vi "{TMPL} MAIN - App.vi"() -> ()   [LabVIEW 2023, in "TLB` InstStu GPlugin Template.lvlib" / "{TMPL} TLB`.lvclass"]
uses:
  {TMPL} TLB`.lvclass
  Application Components/Trigger API/System Trigger.ctl
  State Machine/State.ctl
  Core Components/Error Handler/TLB` Error Handler.lvclass
  Application Components/Configuration/{TMPL} Station Configuration.lvclass
  {TMPL} TLB`.lvclass/{TMPL} TLB`.ctl
  <vilib>/Utility/error.llb/Error Cluster From Error Code.vi
  <vilib>/ErrorRing/Error Ring.xnode
  Application Components/Trigger API/{TMPL} Trigger API.lvlib
  TLB` InstStu GPlugin Template.lvlib
  Core Components/Actions/Actions.lvlib
  Core Components/Dependencies/TLB`_Dependencies.lvlib
panel:
  out "top banner":u32(colorbox)=44412
  out "iq graph":waveform(sgl)[](graph) caption="Q Data"
  out "iq graph 2":waveform(sgl)[](graph) caption="Q Data"
  out "iq graph 3":waveform(sgl)[](graph) caption="Q Data"
  out "iq graph 4":waveform(sgl)[](graph) caption="Q Data"
  in  "error":bool
  out "error background":u32(colorbox)=15461355
  in  "settings gear":bool
  in  "connect":bool
  in  "run":bool
  in  "single":bool
  out "title":string="INST STU GPLUGIN`"
  in  "INSTRUMENT":refnum<visa-resource-name>
  out "error out":errorcluster
  in  "digital offset":dbl caption="DIGITAL OFFSET" format="%1_3p"
  in  "digital gain":dbl=-10.0 caption="DIGITAL GAIN" format="%1_3p dB"
  in  "finite records?":bool=TRUE
  in  "iq rate":dbl=2160000000.0 caption="IQ  RATE" format="%1_6p samples/sec"
  in  "no of samples":u64=1000 caption="NO. SAMPLES"
  in  "no of records":u64=25 caption="NO. RECORDS"
  in  "finite samples?":bool=TRUE
  in  "acq sample rate":dbl=2160000000.0 caption="ACQ SAMPLE RATE" format="%1_6p samples/sec"
  out "State":string="<Shutdown> "
  out "Status":string
  # "Section  A"
  # "Section B"
  # "Category A"
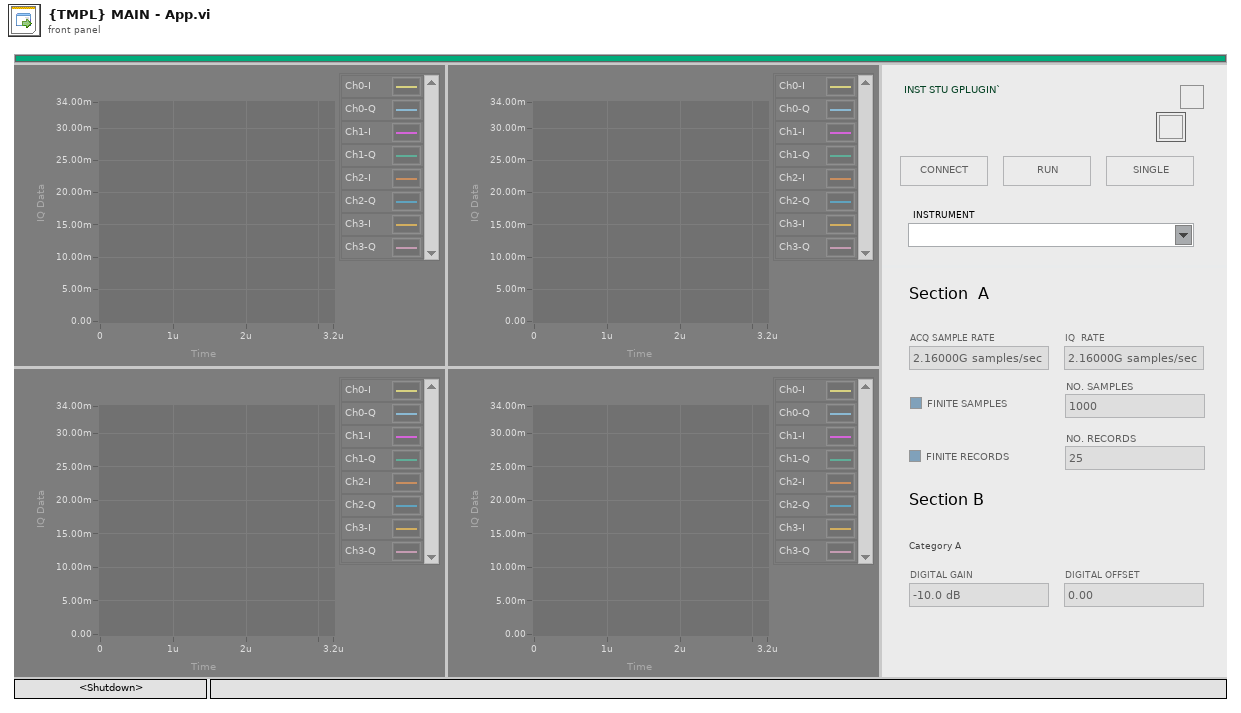
[diagram p1: front panel]
types:
  T1 = typedef "TLB` InstStu GPlugin Template.lvlib/{TMPL} TLB`.lvclass/State.ctl" = enum16{"<Startup>", "Idle", "Connected", "Monitoring", "<Shutdown>", "<Error>"}
  T2 = enum16{"Close Display", "Clear References", "Close Error Handler"}
  T3 = enum16{"Clear SR", "Set Display", "Set Shifter", "Initialize Events", "Init Q"}
  T4 = typedef "TLB` InstStu GPlugin Template.lvlib/{TMPL} Trigger API.lvlib/System Trigger.ctl" = enum16{"<None>", "Connect", "Start Acquisition", "Stop Acquisition", "Disconnect", "Load Configuration", "Save Configuration", "<Return to Safe State Actions>", "<Cache User Parameters>", "<Close Application>", "<Error>"}
  T5 = refnum<class "{TMPL} Station Configuration.lvclass">
  T6 = typedef "TLB` InstStu GPlugin Template.lvlib/_UI CORE Event References.ctl" = cluster{"Exit Event":refnum<user-event>, "State Indicator":refnum<user-event>, "Status Indicator":refnum<user-event>}
  T7 = typedef "TLB` InstStu GPlugin Template.lvlib/_UI APP Event References.ctl" = cluster{"Exit Event":refnum<user-event>}
  T8 = enum32{"Invalid", "Standard", "Closed", "Hidden", "Minimized", "Maximized"}
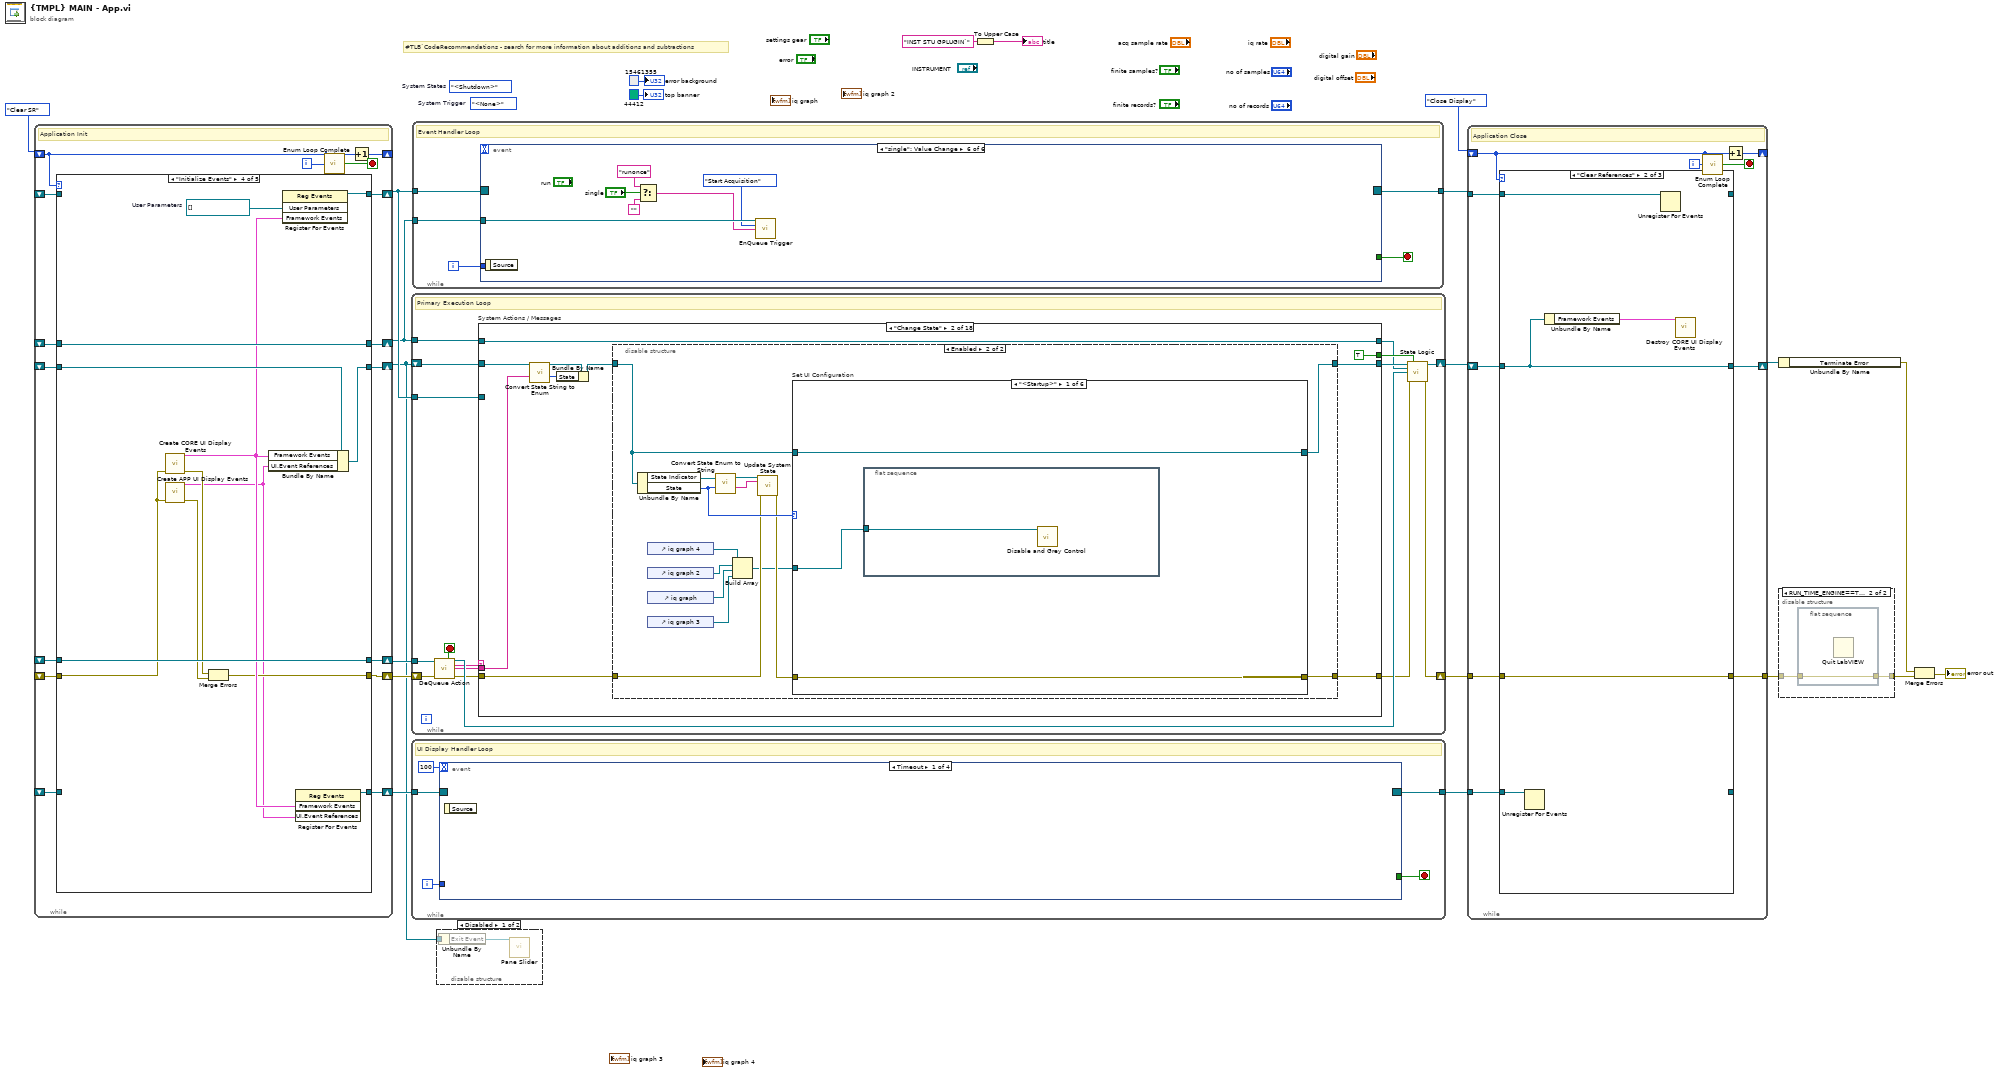
[diagram p0: block diagram]
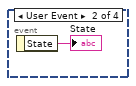
[diagram p3: hidden frame]
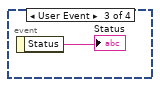
[diagram p4: hidden frame]
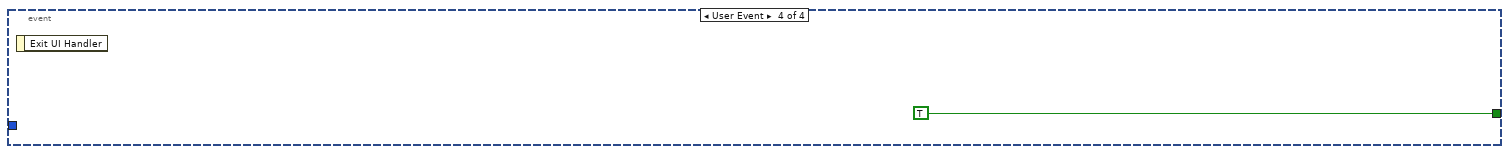
[diagram p5: hidden frame]
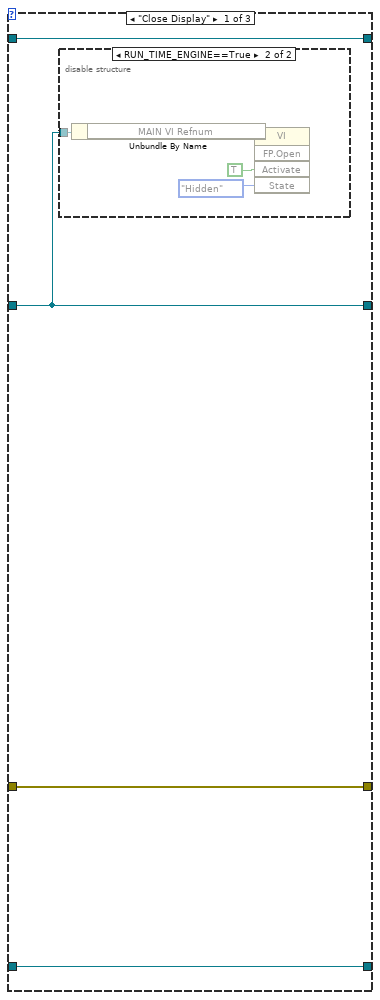
[diagram p7: hidden frame]
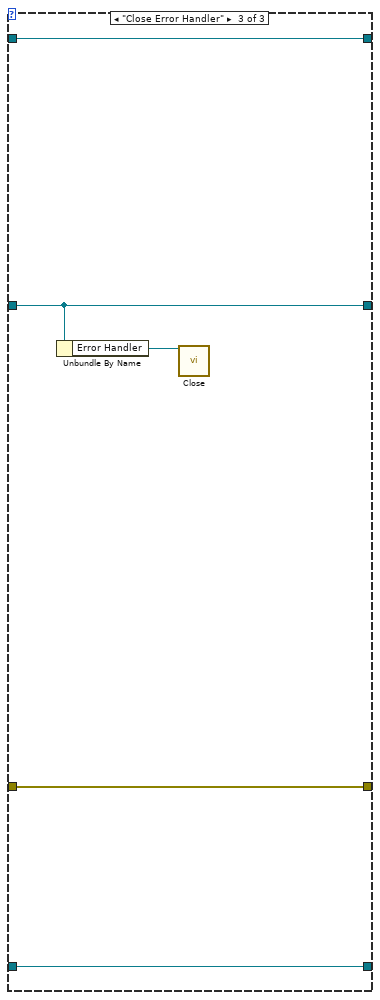
[diagram p9: hidden frame]
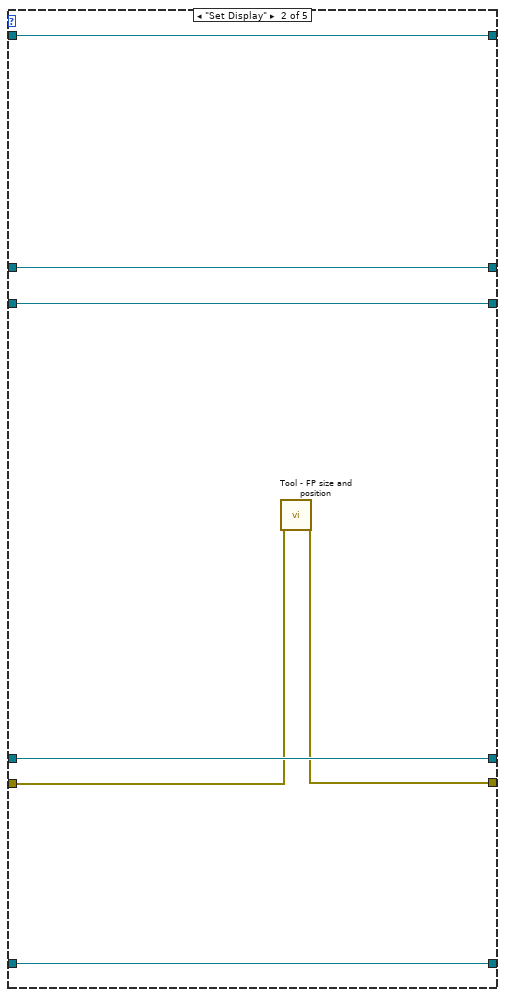
[diagram p11: hidden frame]
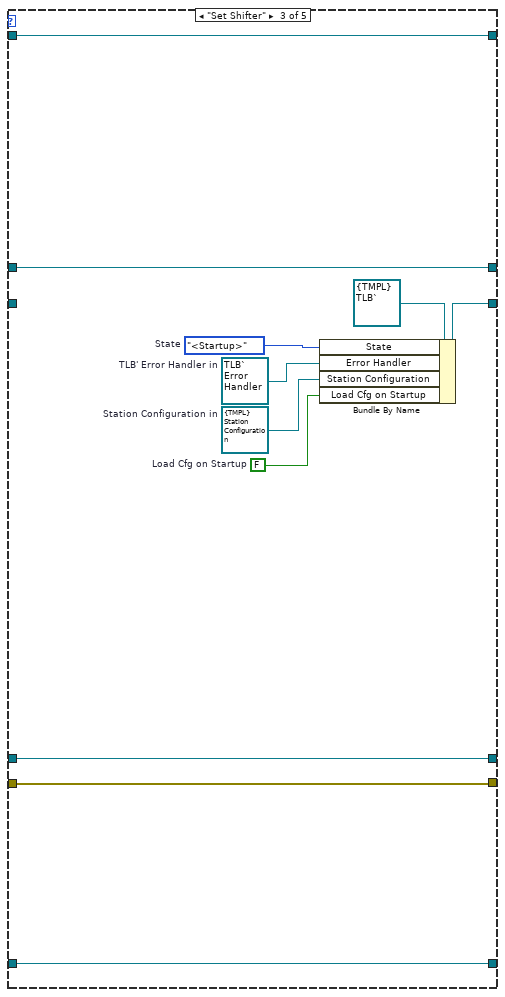
[diagram p12: hidden frame]
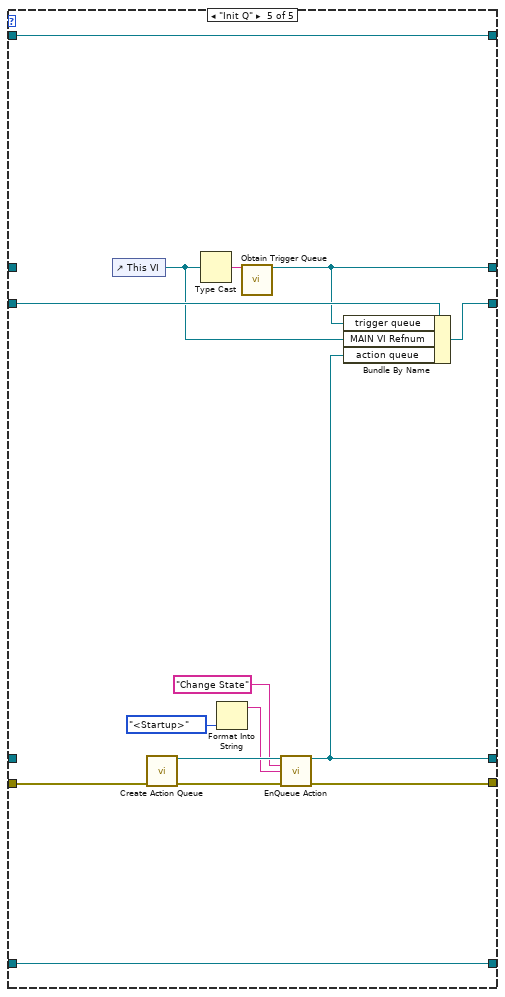
[diagram p13: hidden frame]
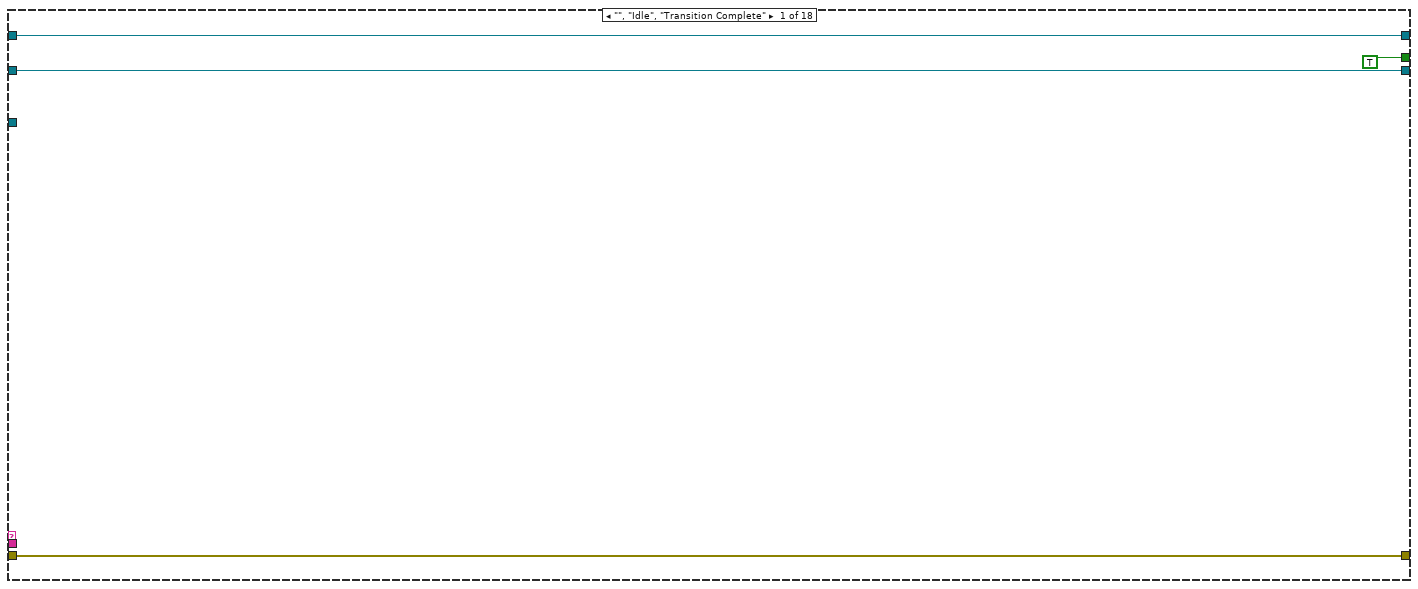
[diagram p14: hidden frame]
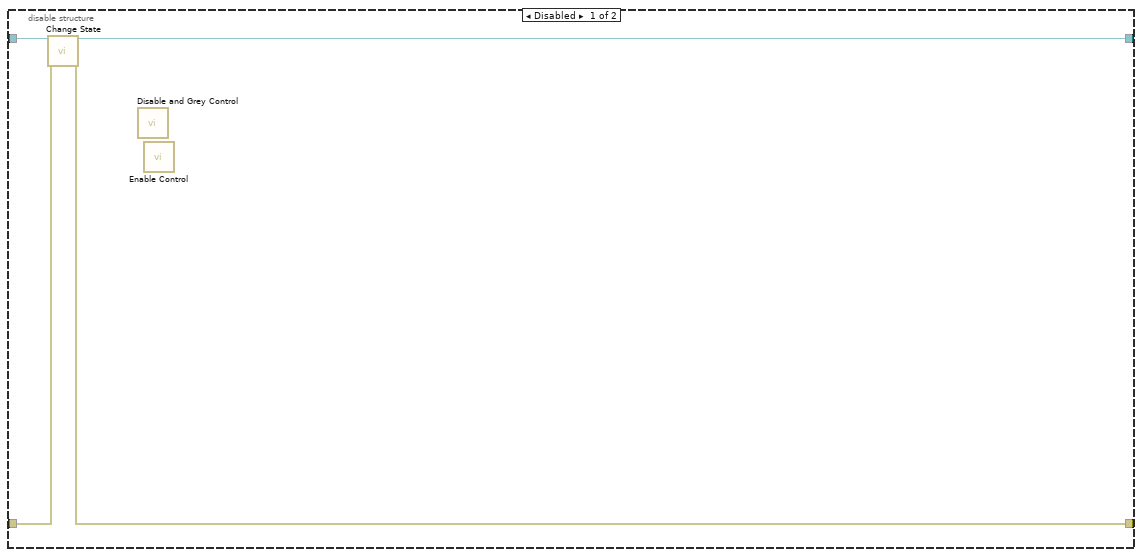
[diagram p15: hidden frame]
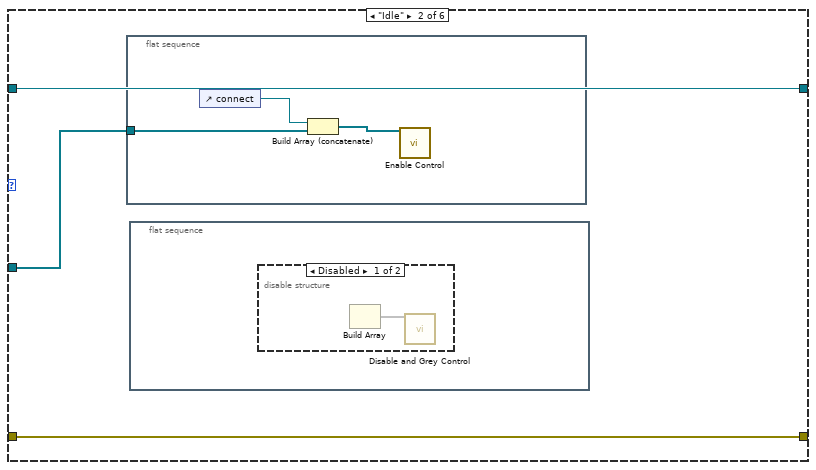
[diagram p16: hidden frame]
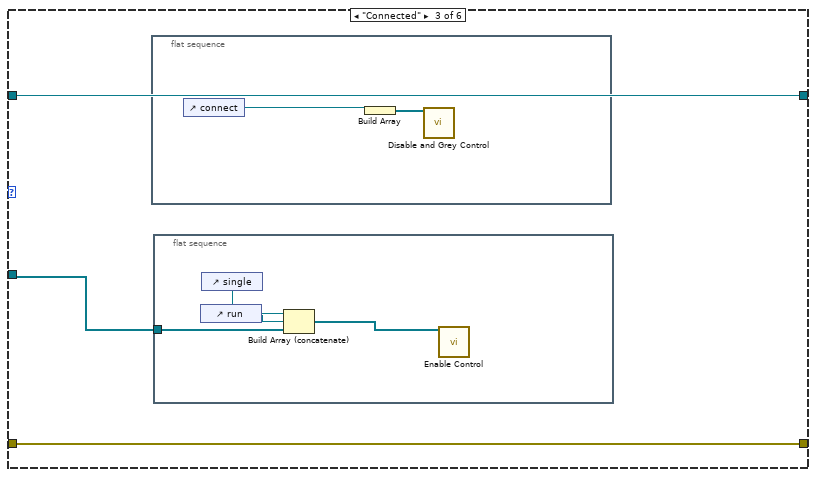
[diagram p18: hidden frame]
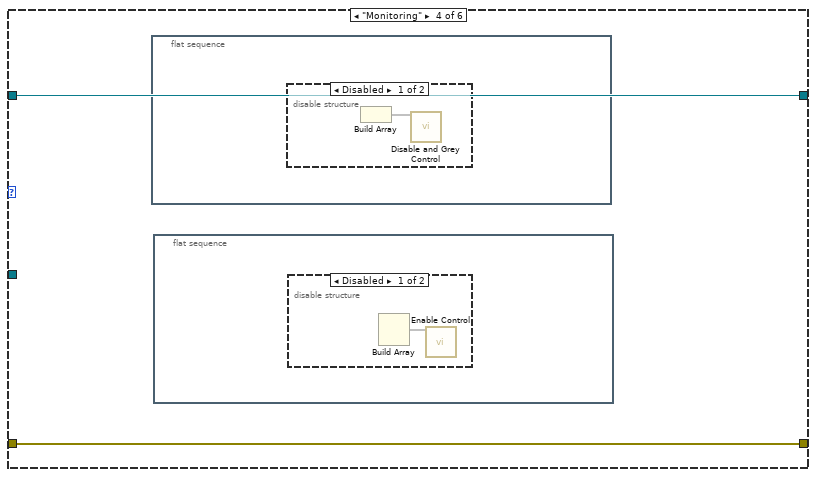
[diagram p19: hidden frame]
diagram:
  (unwired) State."<Shutdown>"  # System States
  (unwired) System_Trigger."<None>"  # System Trigger
  # "#TLB`CodeRecommendations - search for more information about additions and subtractions"
  n1 = while {
    shift-right: [w33] -> _
    shift-left: T3."Clear SR" -> [w22]
    shift-right: [w37] -> w21
    shift-left: _ -> [w32]
    shift-right: [w34] -> w16
    shift-left: _ -> [w31]
    shift-right: [w36] -> w15
    shift-left: _ -> [w30]
    shift-right: [w35] -> w5
    shift-left: _ -> [w29]
    shift-right: [w28] -> w11
    shift-left: _ -> [w27]
    shift-right: [w26] -> w14
    shift-left: _ -> [w25]
    i -> [w23]
    stop <- w24 stop-if-true
    # "Application Init"
    n2 = case shown="\"Initialize Events\"" w22 {
      tunnel: [_ w42 w55 w68 w69] -> w37
      tunnel: [_ w40 w54 w58 w75] -> w34
      tunnel: [_ w44 w50 w66 w81] -> w35
      tunnel: [_ w43 w53 w65 w83] -> w36
      tunnel: w32 -> [_ w42 w55 w68 _]
      tunnel: w31 -> [_ w41 w54 w57 w77]
      tunnel: w30 -> [_ w43 w53 _ w83]
      tunnel: w29 -> [_ w44 _ w67 w82]
      tunnel: [_ w39 w52 w64 w70] -> w28
      tunnel: w27 -> [_ w39 w52 w64 _]
      tunnel: [_ w38 w48 w62 w78] -> w26
      tunnel: w25 -> [_ w38 w48 _ w78]
      frame "Clear SR" {
      }
      frame "Set Display" {
        n3 = call "Tool - FP size and position.vi"("error in (no error)"=w41) -> ("error out"=w40:errorcluster)  [unwired: 17 in, 1 out]
      }
      frame "Set Shifter" {
        w45 = FALSE  # Load Cfg on Startup
        w46 = T5 refnum  # Station Configuration in
        w47 = refnum<class "TLB` Error Handler.lvclass"> refnum  # TLB' Error Handler in
        w51 = State."<Startup>"  # State
        n4 = Bundle By Name(cluster=refnum<class "{TMPL} TLB`.lvclass"> refnum ("TLB` Template.lvlib:TLB' Template.lvclass"), "State"=w51, "Error Handler"=w47, "Station Configuration"=w46, "Load Cfg on Startup"=w45) -> (w50:refnum<class "{TMPL} TLB`.lvclass">)
      }
      frame "Initialize Events" {
        w63 = refnum<vi>[] []  # User Parameters
        n5 = call "Create CORE UI Display Events.vi"("error in"=w57) -> ("Framework Events"=w61:T6, "error out"=w60:errorcluster)  [unwired: 13 in]
        n6 = call "Create APP UI Display Events.vi"("error in"=w57) -> ("UI.Event References"=w56:T7, "error out"=w59:errorcluster)  [unwired: 13 in]
        n7 = Merge Errors(w60, w59) -> (w58:errorcluster)
        n8 = Bundle By Name(cluster=w67, "Framework Events"=w61, "UI.Event References"=w56) -> (w66:refnum<class "{TMPL} TLB`.lvclass">)
        n9 = register-events(w63, w61) -> (reference out=w65:refnum<event-registration>)  [unwired: 2 in, 1 out]
        n10 = register-events(w61, w56) -> (reference out=w62:refnum<event-registration>)  [unwired: 2 in, 1 out]
      }
      frame "Init Q" {
        n11 = control-ref of="This VI"() -> (w80:refnum<vi>)
        n12 = call "Create Action Queue.vi"("error in"=w77) -> ("action queue out"=w74:refnum<queue>, "error out"=w76:errorcluster)  [unwired: 13 in]
        n13 = Type Cast(x=w80) -> (*(type *) &x=w71:string)  [unwired: 1 in]
        n14 = Format Into String(State."<Startup>" ("State")) -> (resulting string=w72:string)  [unwired: 3 in, 1 out]
        n15 = call "Obtain Trigger Queue.vi"("trigger queue name"=w71) -> ("trigger queue out"=w70:refnum<queue>)  [unwired: 13 in, 1 out]
        n16 = call "EnQueue Action.vi"("action queue in"=w74, "action"="Change State" ("Message Name"), "data in"=w72, "error in"=w76) -> ("action queue out"=w69:refnum<queue>, "error out"=w75:errorcluster)  [unwired: 10 in]
        n17 = Bundle By Name(cluster=w82, "trigger queue"=w70, "MAIN VI Refnum"=w80, "action queue"=w69) -> (w81:refnum<class "{TMPL} TLB`.lvclass">)
      }
    }
    n18 = call "Enum Loop Complete.vi"("Current State Enum"=w22, "Itteration"=w23) -> ("Loop Complete?"=w24:bool)  [unwired: 12 in, 1 out]
    n19 = Increment(x=w22) -> (x+1=w33:T3)
  }
  n20 = while {
    shift-right: [w94] -> w13
    shift-left: w16 -> [w89]
    shift-right: [w96] -> w17
    shift-left: w5 -> [w98]
    tunnel: w21 -> [w90]
    tunnel: w15 -> [w97]
    tunnel: w11 -> [w93]
    stop <- w88 stop-if-true
    # "Primary Execution Loop"
    n21 = call "DeQueue Action.vi"("action queue in"=w90, "error in"=w89) -> ("exit?"=w88:bool, "action queue out"=w99:refnum<queue>, "action"=w86:string, "action value"=w84:string, "error out"=w87:errorcluster)  [unwired: 8 in, 1 out]
    n22 = case "System Actions / Messages" shown="\"Change State\"" w86 {
      selector: w86 -> [_ _ _ _ _ _ _ _ _ _ _ _ _ _ _ _ _ w264]
      tunnel: [w103 w110 w174 w181 w182 w191 w200 w214 w217 w224 w230 w233 w236 w241 w246 w247 w259 w263] -> w91
      tunnel: w87 -> [w103 w109 w174 w181 w182 w194 w200 w214 w217 w222 w230 w233 w236 w240 w246 w248 w260 _]
      tunnel: w98 -> [w100 w108 w172 w180 w185 w192 w203 w213 w215 w218 w229 w232 w235 w243 w245 w251 w262 w266]
      tunnel: [w100 w104 w175 w180 w184 w197 w206 w213 w215 w219 w229 w232 w235 w243 w245 w250 w261 w266] -> w95
      tunnel: w97 -> [_ _ _ _ _ _ w204 _ _ _ _ _ _ _ _ _ _ _]
      tunnel: [w101 w111 w173 w179 w186 w198 w205 w212 w216 w227 w228 w231 w234 w238 w244 w254 w255 w265] -> w85
      tunnel: w93 -> [w101 w111 w173 w179 w186 w198 w205 w212 w216 w227 w228 w231 w234 w238 w244 w254 w255 w265]
      tunnel: [TRUE TRUE _ _ _ _ _ _ _ _ _ _ _ _ _ _ _ _] -> w92
      tunnel: w84 -> [_ w107 _ _ _ _ _ _ _ _ _ _ _ _ _ _ _ _]
      frame "", "Idle", "Transition Complete" {
      }
      frame "Change State" {
        n23 = call "Convert State String to Enum.vi"("state in"=w107) -> ("state out"=w106:T1)  [unwired: 13 in, 1 out]
        n24 = Bundle By Name(cluster=w108, "State"=w106) -> (w105:refnum<class "{TMPL} TLB`.lvclass">)
        n25 = disable-structure shown="Enabled" {
          disable-tunnel: [w116 w122] -> w110
          disable-tunnel: w109 -> [w115 w123]
          disable-tunnel: w105 -> [w114 w125]
          disable-tunnel: [w113 w124] -> w104
          frame Disabled {
            n26 = call "Change State.vi"("TLB' data in"=w114, "error in"=w115) -> ("TLB' data out"=w113:refnum<class "{TMPL} TLB`.lvclass">, "error out"=w116:errorcluster)  [unwired: 12 in]
            n27 = call "Disable and Grey Control.vi"() -> ()  [unwired: 15 in, 1 out]
            n28 = call "Enable Control.vi"() -> ()  [unwired: 15 in, 1 out]
          }
          frame Enabled {
            n29 = Unbundle By Name(w125) -> ("State Indicator"=w126:refnum<user-event>, "State"=w129:T1)
            n30 = control-ref of="iq graph 4"() -> (w121:refnum<vi>)
            n31 = control-ref of="iq graph 2"() -> (w120:refnum<vi>)
            n32 = control-ref of="iq graph"() -> (w119:refnum<vi>)
            n33 = control-ref of="iq graph 3"() -> (w118:refnum<vi>)
            n34 = call "Convert State Enum to String.vi"("state in"=w129) -> ("state out"=w127:string)  [unwired: 13 in, 1 out]
            n35 = Build Array(w121, w120, w119, w118) -> (w117:refnum<vi>[])
            n36 = call "Update System State.vi"("State Indicator"=w126, "system state message"=w127, "error in"=w123) -> ("error out"=w128:errorcluster)  [unwired: 12 in]
            n37 = case "Set UI Configuration" shown="\"<Startup>\"" w129 {
              tunnel: [w131 w136 w146 w154 w165 w170] -> w122
              tunnel: w128 -> [w131 w136 w146 w154 w165 w170]
              tunnel: [w132 w135 w145 w153 w164 w171] -> w124
              tunnel: w125 -> [w132 w135 w145 w153 w164 w171]
              tunnel: w117 -> [w130 w134 w144 _ w163 _]
              frame "<Startup>" {
                n38 = flat-sequence {
                  tunnel: w130 -> [w133]
                  frame #0 {
                    n39 = call "Disable and Grey Control.vi"("Control Ref"=w133) -> ()  [unwired: 14 in, 1 out]
                  }
                }
              }
              frame "Idle" {
                n40 = flat-sequence {
                  tunnel: w134 -> [w143]
                  frame #0 {
                    n41 = control-ref of="connect"() -> (w141:refnum<vi>)
                    n42 = Build Array (concatenate)(w141, w143) -> (w142:refnum<vi>[])
                    n43 = call "Enable Control.vi"("Control Ref"=w142) -> ()  [unwired: 14 in, 1 out]
                  }
                }
                n44 = flat-sequence {
                  frame #0 {
                    n45 = disable-structure shown="Disabled" {
                      frame Disabled {
                        n46 = Build Array() -> (w137:void[], w140:dbl, w139:dbl, w138:dbl)
                        n47 = call "Disable and Grey Control.vi"("Control Ref"=w137) -> ()  [unwired: 14 in, 1 out]
                      }
                      frame Enabled {
                      }
                    }
                  }
                }
              }
              frame "Connected" {
                n48 = flat-sequence {
                  frame #0 {
                    n49 = control-ref of="connect"() -> (w152:refnum<vi>)
                    n50 = Build Array(w152) -> (w151:refnum<vi>[])
                    n51 = call "Disable and Grey Control.vi"("Control Ref"=w151) -> ()  [unwired: 14 in, 1 out]
                  }
                }
                n52 = flat-sequence {
                  tunnel: w144 -> [w150]
                  frame #0 {
                    n53 = control-ref of="run"() -> (w147:refnum<vi>)
                    n54 = control-ref of="single"() -> (w148:refnum<vi>)
                    n55 = Build Array (concatenate)(w148, w147, w150) -> (w149:refnum<vi>[])
                    n56 = call "Enable Control.vi"("Control Ref"=w149) -> ()  [unwired: 14 in, 1 out]
                  }
                }
              }
              frame "Monitoring" {
                n57 = flat-sequence {
                  frame #0 {
                    n58 = disable-structure shown="Disabled" {
                      frame Disabled {
                        n59 = Build Array() -> (w161:void[], w162:dbl, w160:dbl)
                        n60 = call "Disable and Grey Control.vi"("Control Ref"=w161) -> ()  [unwired: 14 in, 1 out]
                      }
                      frame Enabled {
                      }
                    }
                  }
                }
                n61 = flat-sequence {
                  frame #0 {
                    n62 = disable-structure shown="Disabled" {
                      frame Disabled {
                        n63 = Build Array() -> (w156:void[], w159:dbl, w155:dbl, w158:dbl, w157:dbl)
                        n64 = call "Enable Control.vi"("Control Ref"=w156) -> ()  [unwired: 14 in, 1 out]
                      }
                      frame Enabled {
                      }
                    }
                  }
                }
              }
              frame "<Shutdown>" {
                n65 = flat-sequence {
                  tunnel: w163 -> [w169]
                  frame #0 {
                    n66 = control-ref of="run"() -> (w166:refnum<vi>)
                    n67 = control-ref of="single"() -> (w167:refnum<vi>)
                    n68 = Build Array (concatenate)(w167, w166, w169) -> (w168:refnum<vi>[])
                    n69 = call "Disable and Grey Control.vi"("Control Ref"=w168) -> ()  [unwired: 14 in, 1 out]
                  }
                }
              }
              frame "<Error>" {
              }
            }
          }
        }
      }
      frame "Cache User Parameters" {
        n70 = disable-structure "<Add Your User Parameter Terminals Here>" shown="Disabled" {
          disable-tunnel: [w177 w178] -> w175
          disable-tunnel: w172 -> [w176 w178]
          frame Disabled {
            n71 = Bundle By Name(cluster=w176) -> (w177:refnum<class "{TMPL} TLB`.lvclass">)  [unwired: 2 in]
          }
          frame Enabled {
          }
        }
      }
      frame "/*********INITialize********/" {
      }
      frame "INIT::Load Application Base Path" {
        n72 = disable-structure shown="Default" {
          disable-tunnel: [w187 w189] -> w183
          frame condition #0 (active) {
            n73 = Current VI's Path() -> (path=w188:path)
            n74 = Strip Path(path=w188) -> (stripped path=w187:path)  [unwired: 1 out]
          }
          frame condition #1 {
            n75 = call <vilib>:"Application Directory.vi"() -> ("Application Directory"=w189:path)
          }
        }
        n76 = Bundle By Name(cluster=w185, "Application Base Path"=w183) -> (w184:refnum<class "{TMPL} TLB`.lvclass">)
      }
      frame "INIT::Initialize Error Handler" {
        n77 = Unbundle By Name(w192) -> ("Application Base Path"=w199:path)
        n78 = Unbundle By Name(w192) -> ("Error Handler"=w193:refnum<class "TLB` Error Handler.lvclass">)
        n79 = Build Path(base path=w199, name or relative path="System Level Errors\\System Errors.txt") -> (appended path=w195:path)
        n80 = call-dynamic "Open.vi"("error handler in"=w193, "error log path in"=w195, "error in"=w194) -> ("error handler out"=w196:refnum<class "TLB` Error Handler.lvclass">, "error out"=w191:errorcluster)  [unwired: 11 in]
        n81 = Bundle By Name(cluster=w192, "Error Handler"=w196) -> (w197:refnum<class "{TMPL} TLB`.lvclass">)
      }
      frame "INIT::Register User Parameters" {
        n82 = disable-structure shown="Enabled" {
          disable-tunnel: [w207 refnum<vi>[] [] ("User Parameter Controls")] -> w202
          frame Disabled {
            n83 = stacked-sequence "Stacked Sequence Structure :: Allows for a lot of controls" {
              tunnel: [w210] -> w207
              frame #0 {
                n84 = Build Array() -> (w210:void[], w209:dbl, w208:dbl)
              }
            }
          }
          frame Enabled {
          }
        }
        n85 = Build Array (concatenate)(w202) -> (w201:refnum<vi>[])
        n86 = register-events(reference=w204, w201) -> ()  [unwired: 2 in, 2 out]
        n87 = Bundle By Name(cluster=w203, "User Parameter Controls"=w201) -> (w206:refnum<class "{TMPL} TLB`.lvclass">)
      }
      frame "INIT::FP Values" {
        # "#TLB`CodeRecommendations - initialize FP values here"
      }
      frame "INIT::Initialize System Parameters" {
      }
      frame "CFG::Load Station Configuration" {
        n88 = Unbundle By Name(w218) -> ("Station Configuration"=w221:T5)
        n89 = Unbundle By Name(w218) -> ("Application Base Path"=w226:path)
        n90 = Build Path(base path=w226, name or relative path="System Configuration\\Station Configuration.ini") -> (appended path=w223:path)
        n91 = call-dynamic "Load Configuration.vi"("INI Station Configuration in"=w221, "INI file path in"=w223, "error in"=w222) -> ("INI Station Configuration out"=w220:T5, "error out"=w224:errorcluster)  [unwired: 11 in]
        n92 = Bundle By Name(cluster=w218, "Station Configuration"=w220) -> (w219:refnum<class "{TMPL} TLB`.lvclass">)
      }
      frame "/*********PRImary EXEcution********/" {
      }
      frame "APP::Update Display" {
      }
      frame "/*********SHUTDOWN********/" {
      }
      frame "Exit" {
        w239 = refnum<class> refnum  # event data
        # "Don't wire 'Error In'\nMust Execute Regardless"
        n93 = Unbundle By Name(w243) -> ("Exit Event"=w237:refnum<user-event>)
        n94 = Generate User Event(user event=w237, event data cluster=w239) -> (error out=w242:errorcluster)  [unwired: 2 in, 1 out]
        n95 = Merge Errors(w240, w242) -> (w241:errorcluster)
      }
      frame "/*********ERRor Handler********/" {
      }
      frame "ERR::Log" {
        n96 = Unbundle By Name(w251) -> ("Error Handler"=w253:refnum<class "TLB` Error Handler.lvclass">)
        n97 = call-dynamic "Log.vi"("error handler in"=w253) -> ("error handler out"=w252:refnum<class "TLB` Error Handler.lvclass">, "error out"=w249:errorcluster)  [unwired: 13 in]
        n98 = Bundle By Name(cluster=w251, "Error Handler"=w252) -> (w250:refnum<class "{TMPL} TLB`.lvclass">)
        n99 = Merge Errors(w248, w249) -> (w247:errorcluster)
      }
      frame "ERR::Dialog" {
        n100 = Unbundle By Name(w262) -> ("Error Handler"=w258:refnum<class "TLB` Error Handler.lvclass">)
        n101 = call-dynamic "Dialog.vi"("error handler in"=w258, "trigger queue in"=w255) -> ("error handler out"=w257:refnum<class "TLB` Error Handler.lvclass">, "error out"=w256:errorcluster)  [unwired: 12 in]
        n102 = Merge Errors(w260, w256) -> (w259:errorcluster)
        n103 = Bundle By Name(cluster=w262, "Error Handler"=w257) -> (w261:refnum<class "{TMPL} TLB`.lvclass">)
      }
      frame Default {
        n104 = xnode "Error Ring"("parameter 0"=w264) -> ("error out"=w263:errorcluster)
      }
    }
    n105 = call "State Logic.vi"("TLB' data in"=w95, "process state logic enable"=w92, "trigger queue in"=w85, "action queue in"=w99, "error in"=w91) -> ("TLB' data out"=w96:refnum<class "{TMPL} TLB`.lvclass">, "error out"=w94:errorcluster)  [unwired: 9 in]
  }
  n106 = while {
    tunnel: w14 -> [w278]
    tunnel: [w274] -> w12
    i -> [w277]
    stop <- w276 stop-if-true
    # "UI Display Handler Loop"
    n107 = event shown="[0] Timeout" {
      selector: w278 -> [_ _ _ _]
      dyn-events: [_ _ _ _] -> w274
      timeout: 100 -> [_ _ _ _]
      tunnel: w277 -> [_ _ _ _]
      tunnel: [_ _ _ TRUE] -> w276
      event Timeout {
        n108 = event-data() -> ()  [unwired: 2 out]
      }
      event User Event {
        n109 = event-data() -> ("State"=→"State":string)  [unwired: 1 out]
      }
      event User Event {
        n110 = event-data() -> ("Status"=→"Status":string)  [unwired: 1 out]
      }
      event User Event {
        n111 = event-data() -> ()  [unwired: 2 out]
      }
    }
  }
  n112 = while {
    tunnel: w15 -> [w285]
    tunnel: [w284] -> w18
    tunnel: w11 -> [w282]
    i -> [w283]
    stop <- w286 stop-if-true
    # "Event Handler Loop"
    n113 = event shown="[5] \"single\": Value Change" {
      selector: w285 -> [_ _ _ _ _ _]
      dyn-events: [_ _ _ _ _ _] -> w284
      timeout: _ -> [_ _ _ _ _ _]
      tunnel: [_ _ TRUE ("NewVal") _ _ _] -> w286
      tunnel: w283 -> [_ _ _ _ _ _]
      tunnel: w282 -> [w287 _ w311 w315 w318 w324]
      event Panel Close? {
        w289 = TRUE  # Discard?
        n114 = event-data() -> ()  [unwired: 2 out]
        n115 = call "EnQueue Trigger.vi"("trigger queue in"=w287, "system trigger"=System_Trigger."<Close Application>" ("System Trigger")) -> ()  [unwired: 12 in, 2 out]
        n116 = event-data("Discard?"=w289) -> ()  [unwired: 1 in, 1 out]
      }
      event "top banner": Mouse Up {
        n117 = event-data() -> ("Button"=w290:u16, "Mods.Double Click"=w291:bool)  [unwired: 1 out]
        n118 = Equal?(x=u16 2, y=w290) -> (x = y?=w293:bool)
        n119 = Compound Arithmetic op=AND(w293, w291) -> (w292:bool)
        n120 = case "Toggle Menu Visibility :: double RIGHT click on logo" shown="True" w292 {
          frame False {
          }
          frame True {
            n121 = First Call?() -> (First Call?: T/F=w299:bool)
            n122 = feedback #1() -> (w297:bool)  [unwired: 1 in]
            n123 = feedback #2() -> (w298:bool)  [unwired: 1 in]
            n124 = case shown="False" w299 {
              tunnel: [w303 w309] -> w301
              tunnel: [w302 w308] -> w300
              tunnel: w298 -> [w305 _]
              tunnel: w297 -> [w304 _]
              tunnel: [w305 TRUE] -> w296
              tunnel: [w304 TRUE] -> w295
              frame False {
                n125 = Not(x=w305) -> (.not. x?=w303:bool)
                n126 = Not(x=w304) -> (.not. x?=w302:bool)
              }
              frame True {
                n127 = property class="VI"() -> ("TB.Visible"=w309:bool, "Front Panel.ShowMenuBar"=w308:bool)  [unwired: 2 in, 2 out]
              }
            }
            n128 = feedback-in #1(w300) -> ()
            n129 = feedback-in #2(w301) -> ()
            n130 = property class="VI"("TB.Visible"=w296, "Front Panel.ShowMenuBar"=w295) -> ()  [unwired: 2 in, 2 out]
          }
        }
      }
      event User Event {
        n131 = event-data() -> ()  [unwired: 2 out]
        n132 = call "EnQueue Trigger.vi"("trigger queue in"=w311, "system trigger"=System_Trigger."<Close Application>" ("System Trigger")) -> ()  [unwired: 12 in, 2 out]
      }
      event Value Change {
        n133 = event-data() -> ()  [unwired: 2 out]
        n134 = call "EnQueue Trigger.vi"("trigger queue in"=w315, "system trigger"=System_Trigger."<Cache User Parameters>" ("System Trigger")) -> ("trigger queue out"=w314:refnum<queue>)  [unwired: 12 in, 1 out]
        n135 = event "use this event case to register a SPEICIFIC 'User Parameter' for a SPECIFIC action" shown="[0] Timeout" {
          selector: _ -> [_]
          dyn-events: _ -> [_]
          timeout: 0 -> [_]
          tunnel: w314 -> [_]
          event Timeout {
            n136 = event-data() -> ()  [unwired: 1 in, 1 out]
          }
        }
      }
      event "connect": Value Change {
        n137 = event-data() -> ()  [unwired: 2 out]
        n138 = call "EnQueue Trigger.vi"("trigger queue in"=w318, "system trigger"=System_Trigger."Connect" ("System Trigger")) -> ()  [unwired: 12 in, 2 out]
      }
      event "single": Value Change {
        n139 = event-data() -> ()  [unwired: 2 out]
        n140 = Select(t="runonce", s="single", f="") -> (s? t:f=w319:string)
        n141 = call "EnQueue Trigger.vi"("trigger queue in"=w324, "system trigger"=System_Trigger."Start Acquisition" ("System Trigger"), "trigger data"=w319) -> ()  [unwired: 11 in, 2 out]
      }
    }
  }
  n142 = disable-structure shown="Disabled" {
    disable-tunnel: w5 -> [w327 _]
    frame Disabled {
      n143 = Unbundle By Name(w327) -> ("Exit Event"=w326:refnum<user-event>)
      n144 = call "Pane Slider.vi"("User Event in"=w326) -> ("Invoke Button"=w325:refnum<vi>)  [unwired: 14 in]
    }
    frame Enabled {
    }
  }
  n145 = To Upper Case(1:"INST STU GPLUGIN`" ("title")) -> (0:→"title":string)
  n146 = while {
    shift-right: [w337] -> _
    shift-left: T2."Close Display" -> [w330]
    tunnel: w18 -> [w335]
    tunnel: w13 -> [w336]
    tunnel: [w333] -> w20
    shift-right: [w332] -> w9
    shift-left: w17 -> [w334]
    tunnel: w12 -> [w331]
    i -> [w328]
    stop <- w329 stop-if-true
    # "Application Close"
    n147 = case shown="\"Clear References\"" w330 {
      tunnel: [w340 w350 w355] -> w333
      tunnel: [w339 w349 w352] -> w332
      tunnel: [w341 _ w354] -> _
      tunnel: w336 -> [w340 w350 w355]
      tunnel: w335 -> [w341 w348 w354]
      tunnel: w334 -> [w339 w349 w352]
      tunnel: w331 -> [w338 w346 w353]
      tunnel: [w338 _ w353] -> _
      frame "Close Display" {
        n148 = disable-structure shown="RUN_TIME_ENGINE==True" {
          disable-tunnel: w339 -> [_ w343]
          frame condition #0 (active) {
          }
          frame condition #1 {
            n149 = Unbundle By Name(w343) -> ("MAIN VI Refnum"=w342:refnum<vi>)
            n150 = invoke class="VI" method="FP.Open"(reference=w342, "Activate"=TRUE ("Activate?"), "State"=T8."Hidden") -> ()  [unwired: 2 in, 5 out]
          }
        }
      }
      frame "Clear References" {
        n151 = Unregister For Events(event registration refnum=w346) -> ()  [unwired: 1 in, 1 out]
        n152 = Unbundle By Name(w349) -> ("Framework Events"=w347:T6)
        n153 = Unregister For Events(event registration refnum=w348) -> ()  [unwired: 1 in, 1 out]
        n154 = call "Destroy CORE UI Display Events.vi"("UI display events in"=w347) -> ()  [unwired: 14 in, 1 out]
      }
      frame "Close Error Handler" {
        n155 = Unbundle By Name(w352) -> ("Error Handler"=w351:refnum<class "TLB` Error Handler.lvclass">)
        n156 = call-dynamic "Close.vi"("error handler in"=w351) -> ()  [unwired: 14 in, 1 out]
      }
    }
    n157 = call "Enum Loop Complete.vi"("Current State Enum"=w330, "Itteration"=w328) -> ("Loop Complete?"=w329:bool)  [unwired: 12 in, 1 out]
    n158 = Increment(x=w330) -> (x+1=w337:T2)
  }
  n159 = disable-structure shown="RUN_TIME_ENGINE==True" {
    disable-tunnel: [w356 w357] -> w7
    disable-tunnel: w20 -> [w356 w358]
    frame condition #0 (active) {
    }
    frame condition #1 {
      n160 = flat-sequence {
        tunnel: [w359] -> w357
        tunnel: w358 -> [w359]
        frame #0 {
          n161 = Quit LabVIEW() -> ()  [unwired: 1 in]
        }
      }
    }
  }
  n162 = Unbundle By Name(w9) -> ("Terminate Error"=w8:errorcluster)
  n163 = Merge Errors(w8, w7) -> (→"error out":errorcluster)
  "top banner" <- u32 44412 ("top banner")
  "error background" <- u32 15461355 ("error background")
